vi "M3102A test reading.vi"() -> ()   [LabVIEW 2020]
uses:
  <vilib>/Keysight_SD1/DAQ/base/DAQread_AIN.vi
  <vilib>/measure/mascope.llb/Amplitude and Levels 1 chan.vi
  <vilib>/measure/NI_MAPro.lvlib
panel:
  in  "nSlot":i32=5
  in  "nChassis":i32=1
  out "low state level":dbl format="%.2g"
  out "high state level":dbl format="%.2g"
  out "Numeric":dbl
  out "Waveform Graph":waveform(dbl)(graph)
  in  "coupling":i32(ring) items=["DC", "AC"]
  in  "impedance":i32(ring)=1 items=["High Z", "50 Ohms"]
  in  "fullscale":dbl=1.0
  in  "nChannel":i32=1
  out "errorOut":errorcluster
  in  "points":i32=100
  # "Scale depend on impedance."
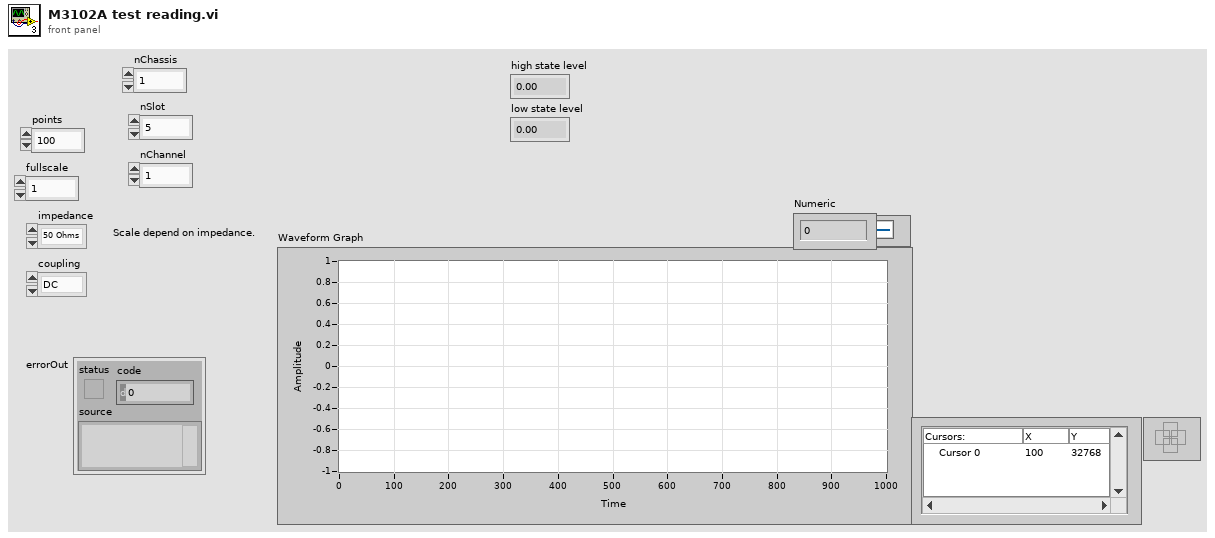
[diagram p1: front panel]
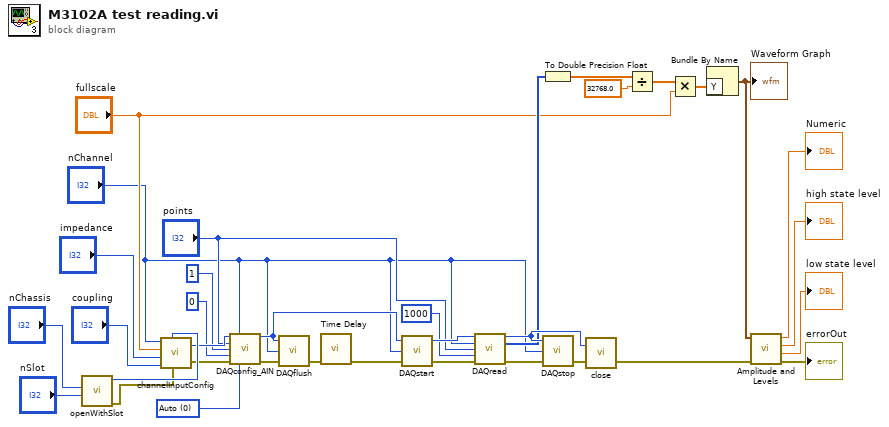
[diagram p0: block diagram]
diagram:
  w26 = 0 items=["Auto", "VI/HVI", "External", "Analog"] ("triggerMode")
  n1 = call <vilib>:"openWithSlot.vi"("nSlot"="nSlot", "nChassis"="nChassis") -> ("errorOut"=w30:errorcluster, "moduleID"=w33:i32)  [unwired: 4 in]
  n2 = call <vilib>:"channelInputConfig.vi"("errorIn"=w30, "moduleID"=w33, "coupling"="coupling", "impedance"="impedance", "fullscale"="fullscale", "nChannel"="nChannel") -> ("errorOut"=w27:errorcluster, "moduleIDout"=w29:i32)
  n3 = call <vilib>:"DAQconfig_AIN.vi"("moduleID"=w29, "nDAQ"="nChannel", "DAQpointsPerCycle"="points", "cycles"=1, "triggerDelay"=0, "errorIn"=w27, "triggerMode"=w26) -> ("moduleIDout"=w12:i32, "errorOut"=w10:errorcluster)  [unwired: 7 in]
  n4 = call <vilib>:"DAQflush.vi"("errorIn"=w10, "nDAQ"="nChannel", "moduleID"=w12) -> ("errorOut"=w9:errorcluster)  [unwired: 1 in, 1 out]
  n5 = call "Time Delay"("error in (no error)"=w9) -> ("error out"=w8:errorcluster)  [unwired: 10 in]
  n6 = call <vilib>:"DAQstart.vi"("errorIn"=w8, "nDAQ"="nChannel", "moduleID"=w12) -> ("errorOut"=w25:errorcluster, "moduleIDout"=w24:i32)  [unwired: 1 in]
  n7 = call-poly <vilib>:"DAQread.vi"("moduleID"=w24, "nDAQ"="nChannel", "DAQpoints"="points", "TimeOut"=1000, "errorIn"=w25) -> ("moduleIDout"=w18:i32, "DAQdata"=w17:i16[], "errorOut"=w21:errorcluster)  [unwired: 8 in]
  n8 = To Double Precision Float(number=w17) -> (double precision float=w16:dbl[])
  n9 = call <vilib>:"DAQstop.vi"("errorIn"=w21, "nDAQ"="nChannel", "moduleID"=w18) -> ("errorOut"=w19:errorcluster)  [unwired: 1 in, 1 out]
  n10 = call <vilib>:"close.vi"("errorIn"=w19, "moduleID"=w18) -> ("errorOut"=w7:errorcluster)  [unwired: 1 in]
  n11 = Divide(x=w16, y=32768.0) -> (x/y=w14:dbl[])
  n12 = Multiply(x=w14, y="fullscale") -> (x*y=w4:dbl[])
  n13 = Bundle By Name("Y"=w4) -> (w1:waveform(dbl))  [unwired: 1 in]
  "Waveform Graph" <- w1
  n14 = call-poly <vilib>:"Amplitude and Levels.vi"("error in (no error)"=w7, "signal in"=w1) -> ("error out"=→"errorOut":errorcluster, "low state level"=→"low state level":dbl, "high state level"=→"high state level":dbl, "amplitude"=→"Numeric":dbl)  [unwired: 6 in]
